vi "read only.vi"() -> ()   [LabVIEW 2015]
panel:
  out "Bus Status":bool
  out "String":string
  out "error out":errorcluster
  in  "stop":bool caption="Press To End Run"
  in  "Desired Bus State":bool
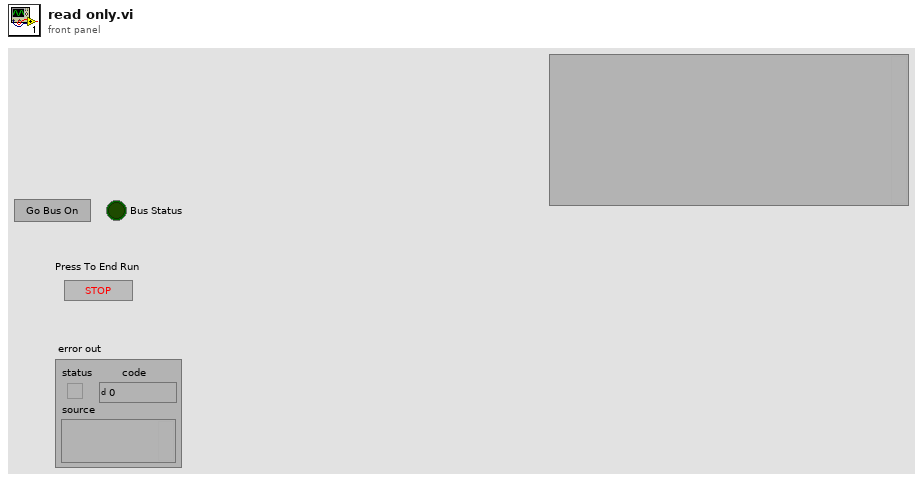
[diagram p1: front panel]
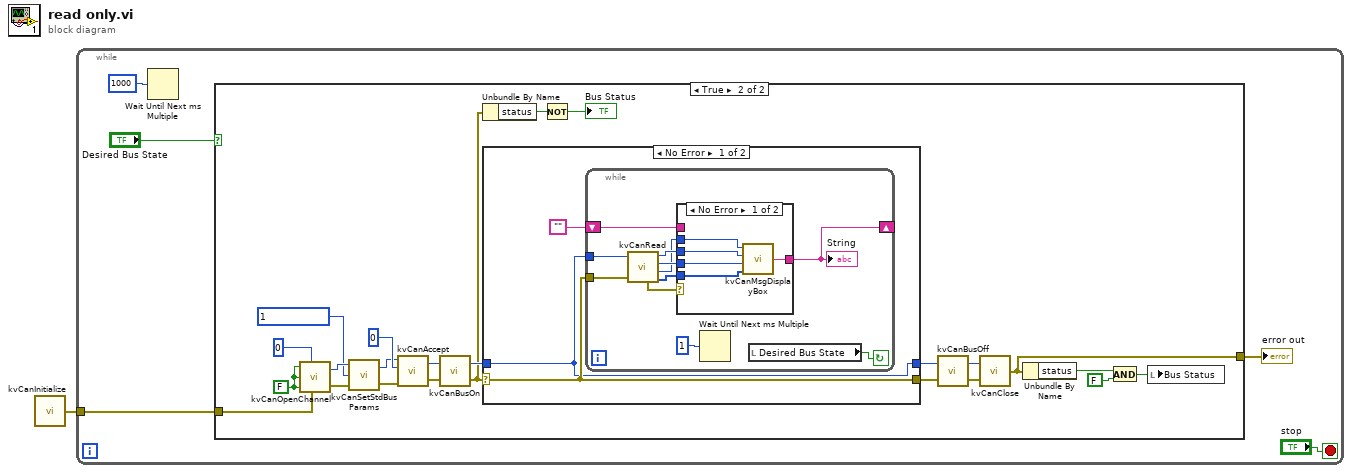
[diagram p0: block diagram]
diagram:
  n1 = call "kvCanInitialize.vi"() -> ("error out (no error)"=w1:errorcluster)
  n2 = while {
    tunnel: w1 -> [w6]
    stop <- "stop" stop-if-true
    n3 = Wait Until Next ms Multiple(millisecond multiple=1000) -> ()  [unwired: 1 out]
    n4 = case shown="True" "Desired Bus State" {
      tunnel: w6 -> [w7 w30]
      tunnel: [w7 w9] -> w5
      frame False {
      }
      frame True {
        w14 = FALSE ("WantExclusive")
        n5 = call "kvCanOpenChannel.vi"("WantExclusive"=w14, "CAN Channel Number"=0, "WantExtended"=w14, "WantVirtual"=w14, "error in (no error)"=w30) -> ("Opened Channel Handle\n(output only)"=w20:i32, "error out"=w19:errorcluster)
        n6 = call "kvCanSetStdBusParams.vi"("error in (no error)"=w19, "Standard CAN Baud Rate"=1 ("Baud Rate"), "Channel Handle (input only)"=w20) -> ("error out"=w18:errorcluster, "Channel Handle (ouput only)"=w17:i32)
        n7 = call "kvCanAccept.vi"("error in (no error)"=w18, "Envelope Mask or Code"=0, "Channel Handle (input only)"=w17) -> ("error out"=w12:errorcluster, "Channel Handle (ouput only)"=w13:i32)  [unwired: 1 in]
        n8 = call "kvCanBusOn.vi"("error in (no error)"=w12, "Channel Handle (input only)"=w13) -> ("error out"=w11:errorcluster, "Channel Handle (ouput only)"=w26:i32)
        n9 = Unbundle By Name(w11) -> ("status"=w10:bool)
        n10 = case shown="No Error" w11 {
          selector: w11 -> [w32 w52]
          tunnel: [w32 w52] -> w22
          tunnel: w26 -> [w31 w51]
          tunnel: [w31 w51] -> w23
          frame No Error {
            n11 = while {
              shift-right: [w40] -> _
              shift-left: "" -> [w41]
              tunnel: w31 -> [w43]
              tunnel: w32 -> [w35]
              stop <- w44 continue-if-true
              n12 = call "kvCanRead.vi"("error in (no error)"=w35, "Channel Handle (input only)"=w43) -> ("Message Data"=w39:u8[], "error out"=w42:errorcluster, "Message Timestamp"=w36:u32, "Message Flags"=w38:u32, "Message Id"=w37:i32)  [unwired: 1 in, 1 out]
              n13 = case shown="No Error" w42 {
                tunnel: w41 -> [_ w50]
                tunnel: [w49 w50] -> w40
                tunnel: w39 -> [w48 _]
                tunnel: w38 -> [w47 _]
                tunnel: w37 -> [w46 _]
                tunnel: w36 -> [w45 _]
                frame No Error {
                  n14 = call "kvCanMsgDisplayBox.vi"("Message Data"=w48, "Message Flags"=w47, "Message Id"=w46, "Time Stamp"=w45) -> ("Output String"=w49:string)
                }
                frame Error {
                }
              }
              "String" <- w40
              n15 = Wait Until Next ms Multiple(millisecond multiple=u32 1) -> ()  [unwired: 1 out]
              n16 = local read "Desired Bus State"() -> (w44:bool)
            }
          }
          frame Error {
          }
        }
        n17 = Not(x=w10) -> (.not. x?=→"Bus Status":bool)
        n18 = call "kvCanBusOff.vi"("error in (no error)"=w22, "Channel Handle (input only)"=w23) -> ("error out"=w24:errorcluster, "Channel Handle (ouput only)"=w25:i32)
        n19 = call "kvCanClose.vi"("error in (no error)"=w24, "Channel Handle (input only)"=w25) -> ("error out"=w9:errorcluster)
        n20 = Unbundle By Name(w9) -> ("status"=w8:bool)
        n21 = And(x=w8, y=FALSE) -> (x .and. y?=w28:bool)
        n22 = local write "Bus Status"(w28) -> ()
      }
    }
    "error out" <- w5
  }
